vi "Read Sequence.vi"(8 "error in (no error)":errorcluster, 9 "Channel Mask":u64, 10 "Config Data":T3, 11 "Connection Data In":T2) -> (0 "error out":errorcluster, 1 "Adquisition Data Out":T1, 3 "Connection Data Out":T2)   [LabVIEW 2014, in "MSX-E3701_dll.lvlib"]
doc: "Recibe el Channel mask y el Config data. Abre el puerto e inicia la adquisición de valores en forma secuencial. Al mismo tiempo lee el estado de las I/O."
uses:
  MSX-E3701_dll.lvlib
  Typedef/Config Data.ctl
  Typedef/Connection Data.ctl
  E:/Repositorio Magnis/INF002/v0/Modules/HAL/Drivers/Sync/ADDI-DATA MSX-E3701/API/MX370x.dll
  MX370x.dll
  E:/Repositorio Magnis/INF002/v0/Modules/HAL/Drivers/Sync/ADDI-DATA MSX-E3701/API/MXCommon.dll
  MXCommon.dll
  Typedef/Adquisition Data.ctl
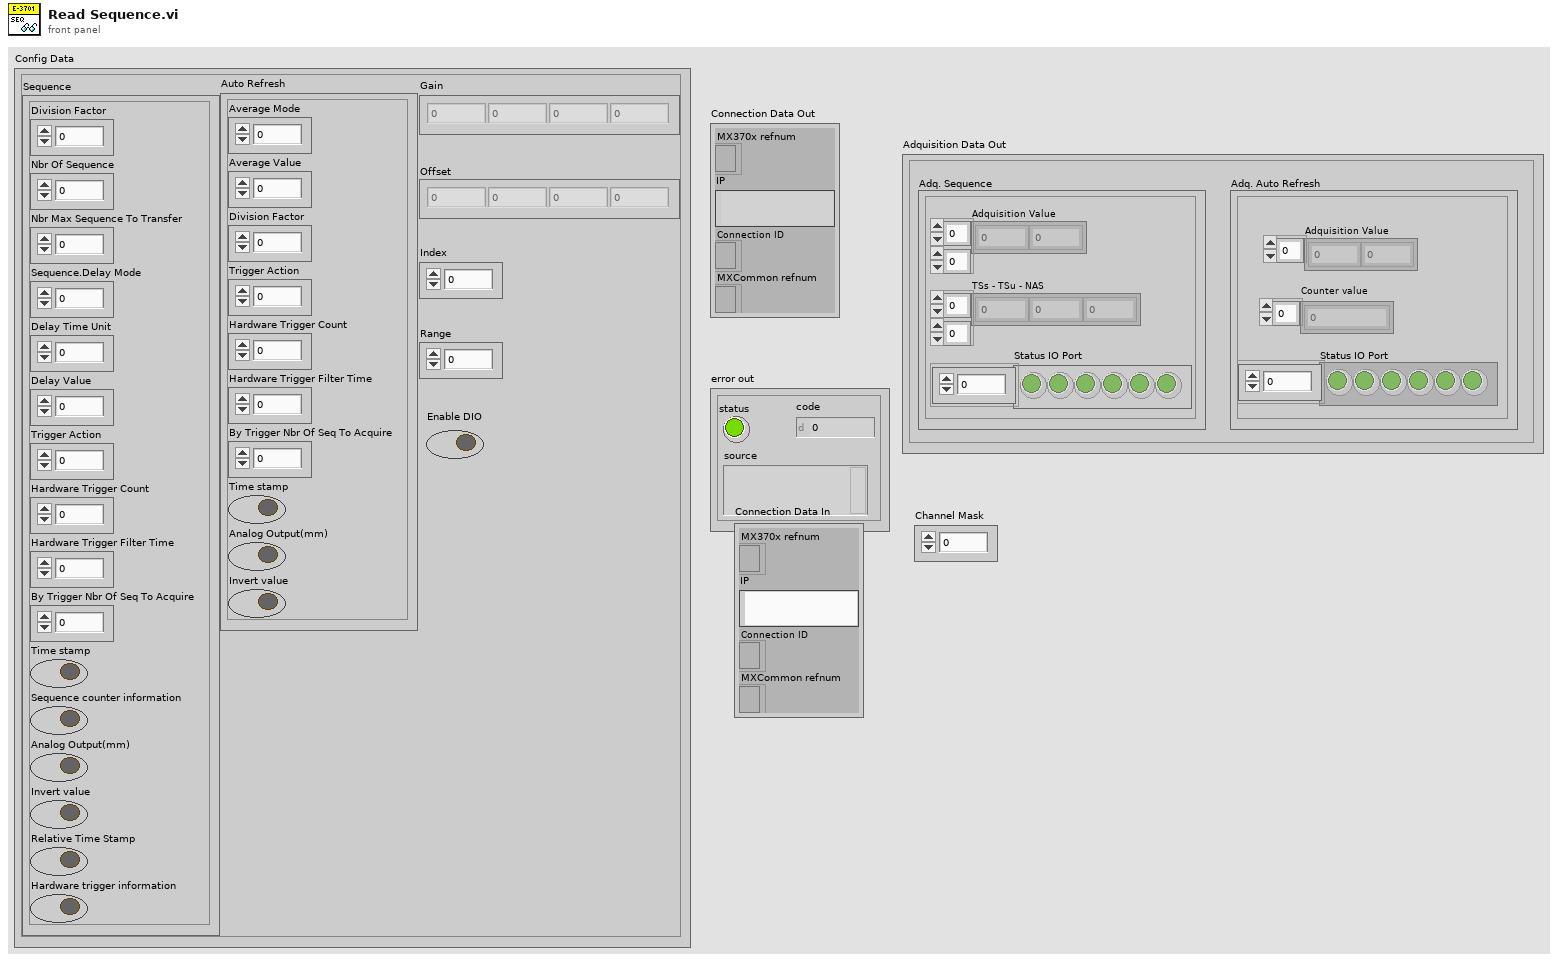
[diagram p1: front panel]
types:
  T1 = typedef "MSX-E3701_dll.lvlib/Adquisition Data.ctl" = cluster{"Adq. Sequence":cluster{"TSs - TSu - NAS":u64[][], "Adquisition Value":u32[][], "Status IO Port":bool[]}, "Adq. Auto Refresh":cluster{"Adquisition Value":u64[], "Status IO Port":bool[], "Counter value":u64[]}}
  T2 = typedef "MSX-E3701_dll.lvlib/Connection Data.ctl" = cluster{"MX370x refnum":refnum<k24>, "IP":string, "Connection ID ":refnum<k5>, "MXCommon refnum":refnum<k24>}
  T3 = typedef "MSX-E3701_dll.lvlib/Config Data.ctl" = cluster{"Auto Refresh":cluster{"Average Mode":u64, "Average Value":u64, "Division Factor":u64, "Trigger Action":u64, "Hardware Trigger Count":u64, "Hardware Trigger Filter Time":u64, "By Trigger Nbr Of Seq To Acquire":u64, "Time stamp":bool, "Analog Output(mm)":bool, "Invert value":bool}, "Gain":sgl[], "Offset":sgl[], "Index":u64, "Range":sgl, "Sequence":cluster{"Division Factor":u64, "Nbr Of Sequence":u64, "Nbr Max Sequence To Transfer":u64, "Sequence.Delay Mode":u64, "Delay Time Unit":u64, "Delay Value":u64, "Trigger Action":u64, "Hardware Trigger Count":u64, "Hardware Trigger Filter Time":u64, "By Trigger Nbr Of Seq To Acquire":u64, "Time stamp":bool, "Sequence counter information":bool, "Analog Output(mm)":bool, "Invert value":bool, "Relative Time Stamp":bool, "Hardware trigger information":bool}, "Enable DIO":bool}
  T4 = cluster{"Division Factor":u64, "Nbr Of Sequence":u64, "Nbr Max Sequence To Transfer":u64, "Sequence.Delay Mode":u64, "Delay Time Unit":u64, "Delay Value":u64, "Trigger Action":u64, "Hardware Trigger Count":u64, "Hardware Trigger Filter Time":u64, "By Trigger Nbr Of Seq To Acquire":u64, "Time stamp":bool, "Sequence counter information":bool, "Analog Output(mm)":bool, "Invert value":bool, "Relative Time Stamp":bool, "Hardware trigger information":bool}
  T5 = enum16{"big-endian, network order", "native, host order", "little-endian"}
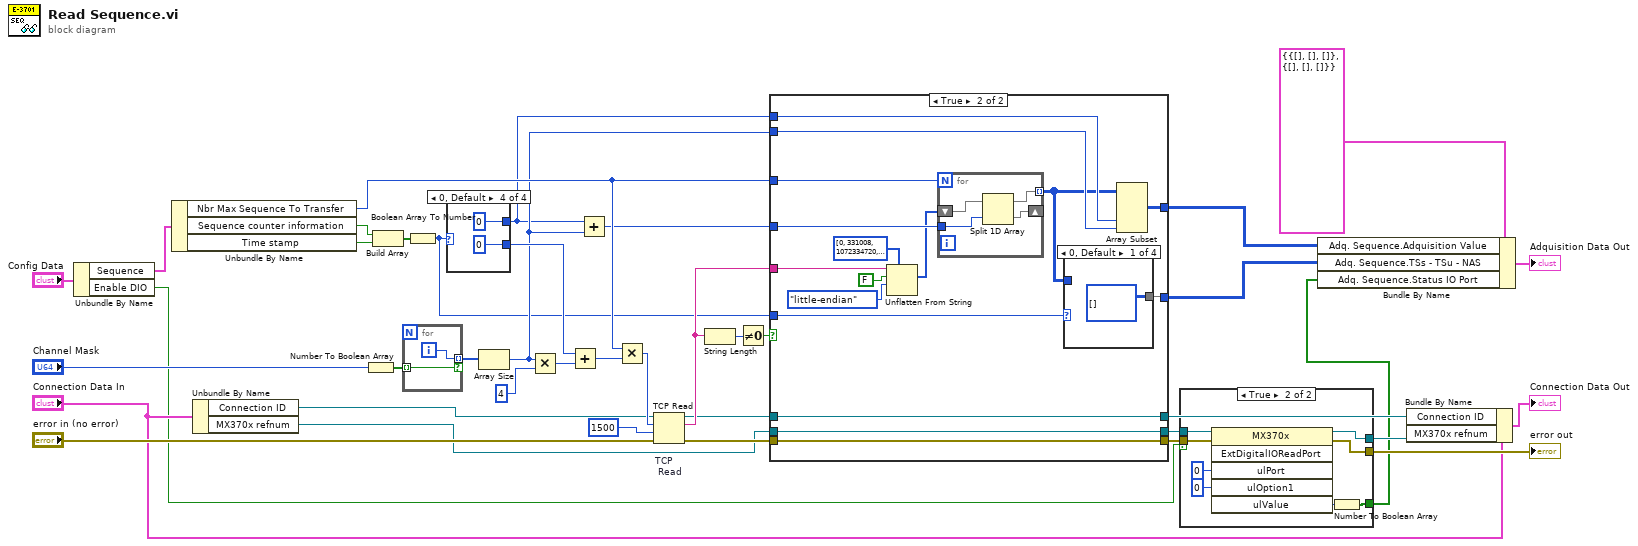
[diagram p0: block diagram]
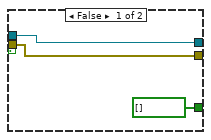
[diagram p2: hidden frame]
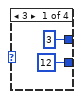
[diagram p3: hidden frame]
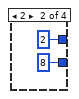
[diagram p4: hidden frame]
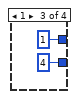
[diagram p5: hidden frame]
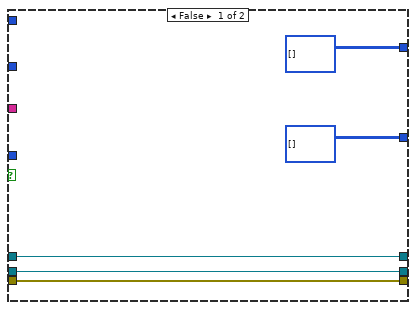
[diagram p6: hidden frame]
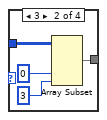
[diagram p7: hidden frame]
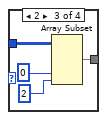
[diagram p8: hidden frame]
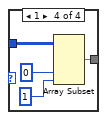
[diagram p9: hidden frame]
diagram:
  n1 = Unbundle By Name("Config Data") -> ("Sequence"=w37:T4, "Enable DIO"=w1:bool)
  n2 = Unbundle By Name(w37) -> ("Nbr Max Sequence To Transfer"=w14:u64, "Sequence counter information"=w13:bool, "Time stamp"=w12:bool)
  n3 = Unbundle By Name("Connection Data In") -> ("Connection ID"=w34:refnum<k5>, "MX370x refnum"=w18:refnum<k24>)
  n4 = Number To Boolean Array(number="Channel Mask") -> (Boolean array=w39:bool[])
  n5 = Build Array(w13, w12) -> (w11:bool[])
  n6 = for {
    tunnel: [w42] -> w38 mode=indexing if=w41
    tunnel: w39 -> [w41] mode=indexing
    i -> [w42]
  }
  n7 = Boolean Array To Number(Boolean array=w11) -> (number=w5:u32)
  n8 = case shown="0, Default" w5 {
    tunnel: [12 8 4 0] -> w10
    tunnel: [3 2 1 0] -> w7
    frame 3 {
    }
    frame 2 {
    }
    frame 1 {
    }
    frame 0, Default {
    }
  }
  n9 = Array Size(array=w38) -> (size(s)=w8:i32)
  n10 = Multiply(x=w8, y=4) -> (x*y=w6:i32)
  n11 = Add(x=w10, y=w6) -> (x+y=w36:i32)
  n12 = Add(x=w7, y=w8) -> (x+y=w9:i32)
  n13 = Multiply(x=w14, y=w36) -> (x*y=w35:u64)
  n14 = TCP Read "TCP\n Read"(connection ID=w34, bytes to read=w35, error in (no error)="error in (no error)", 9:1500 ("timeout ms (25000)")) -> (connection ID out=w21:refnum<k5>, data out=w26:string, error out=w25:errorcluster)  [unwired: 1 in]
  n15 = String Length(string=w26) -> (length=w28:i32)
  n16 = Not Equal To 0?(x=w28) -> (x != 0?=w27:bool)
  n17 = case shown="True" w27 {
    tunnel: w26 -> [_ w69]
    tunnel: w25 -> [w55 w68]
    tunnel: [w55 w68] -> w24
    tunnel: w14 -> [_ w56]
    tunnel: w9 -> [_ w67]
    tunnel: [w54 w66] -> w22
    tunnel: w21 -> [w54 w66]
    tunnel: w18 -> [w53 w65]
    tunnel: [w53 w65] -> w19
    tunnel: [u32[][] [] w64] -> w17
    tunnel: [u32[][] [] w60] -> w16
    tunnel: w8 -> [_ w62]
    tunnel: w7 -> [_ w61]
    tunnel: w5 -> [_ w58]
    frame False {
    }
    frame True {
      n18 = Unflatten From String(type=u32[] [0, 331008, 1072334720, 3195303168, 4729, 331808, 1072334336, 3195309312, 4729, 332608, 1072334080, 3195300096, 4729, 333408, 1072334400, 3195303936, 4729, 334208, 1072334336, 3195305728, 4729, 335008, 1072334400, 3195309568, 4729, 335808, 1072334912, 3195305472, 4729, 336608, 1072333568, 3195304704, 4729, 337408, 1072333440, 3195311872, 4729, 338208, 1072334720, 3195307264, 4729, 339008, 1072334272, 3195311616, 4729, 339808, 1072334272, 3195305984, 4729, 340608, 1072334400, 3195307776, 4729, 341408, 1072334080, 3195308288, 4729, 342208, 1072334720, 3195304448, 4729, 343008, 1072335488, 3195307264, 4729, 343808, 1072334080, 3195302912, 4729, 344608, 1072334272, 3195311360, 4729, 345408, 1072334848, 3195309056, 4729, 346208, 1072334784, 3195301376, 4729, 347008, 1072335168, 3195305472, 4729, 347808, 1072334912, 3195314688, 4729, 348608, 1072334080, 3195299584, 4729, 349408, 1072334144, 3195304448, 4729, 350208, 1072334400, 3195304448, 4729, 351008, 1072335296, 3195304960, 4729, 351808, 1072334144, 3195309824, 4729, 352608, 1072334784, 3195303168, 4729, 353408, 1072334464, 3195305472, 4729, 354208, 1072335168, 3195313920, 4729, 355008, 1072334400, 3195304960, 4729, 355808, 1072334144, 3195304192, 4729, 356608, 1072334528, 3195307776, 4729, 357408, 1072335104, 3195309056, 4729, 358208, 1072333824, 3195308544, 4729, 359008, 1072334208, 3195309312, 4729, 359808, 1072334272, 3195306240, 4729, 360608, 1072334848, 3195309312, 4729, 361408, 1072334656, 3195302912, 4729, 362208, 1072334528, 3195305216, 4729, 363008, 1072334528, 3195304192, 4729, 363808, 1072335232, 3195316480, 4729, 364608, 1072334784, 3195305216, 4729, 365408, 1072333824, 3195308800, 4729, 366208, 1072334784, 3195309312, 4729, 367008, 1072334784, 3195302656, 4729, 367808, 1072333632, 3195310336, 4729, 368608, 1072333568, 3195305984, 4729, 369408, 1072334336, 3195305728, 4729, 370208, 1072334656, 3195304448, 4729, 371008, 1072334208, 3195305984, 4729, 371808, 1072334336, 3195306240, 4729, 372608, 1072334144, 3195302656, 4729, 373408, 1072334592, 3195300864, 4729, 374208, 1072334016, 3195302400, 4729, 375008, 1072334144, 3195307264, 4729, 375808, 1072334528, 3195312640, 4729, 376608, 1072334784, 3195302400, 4729, 377408, 1072333696, 3195305728, 4729, 378208, 1072334656, 3195302144, 4729, 379008, 1072334464, 3195306752, 4729, 379808, 1072334272, 3195306496, 4729, 380608, 1072334272, 3195307776, 4729, 381408, 1072334400, 3195306496, 4729, 382208, 1072334592, 3195300608, 4729, 383008, 1072334400, 3195303168, 4729, 383808, 1072334016, 3195304192, 4729, 384608, 1072334016, 3195309568, 4729, 385408, 1072334912, 3195306496, 4729, 386208, 1072334656, 3195303424, 4729, 387008, 1072334080, 3195302912, 4729, 387808, 1072334592, 3195309312, 4729, 388608, 1072334272, 3195299072, 4729, 389408, 1072334144, 3195304704, 4729, 390208, 1072334272, 3195304960, 4729, 391008, 1072334144, 3195305472, 4729, 391808, 1072334336, 3195301632, 4729, 392608, 1072334464, 3195307008, 4729, 393408, 1072334016, 3195311616, 4729, 394208, 1072335168, 3195310336, 4729, 395008, 1072335232, 3195308288, 4729, 395808, 1072334592, 3195303680, 4729, 396608, 1072334016, 3195308288, 4729, 397408, 1072335296, 3195304448, 4729, 398208, 1072334400, 3195310080, 4729, 399008, 1072334464, 3195302912, 4729, 399808, 1072334848, 3195305728, 4729, 400608, 1072334464, 3195306752, 4729, 401408, 1072334272, 3195306240, 4729, 402208, 1072334656, 3195305216, 4729, 403008, 1072334272, 3195307008, 4729, 403808, 1072335296, 3195315968, 4729, 404608, 1072334336, 3195302656, 4729, 405408, 1072334336, 3195304192, 4729, 406208, 1072334528, 3195309568, 4729, 407008, 1072334912, 3195303168, 4729, 407808, 1072333952, 3195309312, 4729, 408608, 1072334272, 3195307520, 4729, 409408, 1072334464, 3195306496, 4729, 410208, 1072334400, 3195305472] ("Array - Numeric"), binary string=w69, data includes array or string size? (T)=FALSE, byte order (0:big-endian, network order)=T5."little-endian") -> (value=w63:u32[])  [unwired: 1 in, 2 out]
      n19 = for {
        N: w56 -> [_]
        shift-right: [w85] -> _
        shift-left: w63 -> [w88]
        tunnel: [w87] -> w59 mode=indexing
        tunnel: w67 -> [w86]
        n20 = Split 1D Array(array=w88, index=w86) -> (first subarray=w87:u32[], second subarray=w85:u32[])
      }
      n21 = case shown="0, Default" w58 {
        tunnel: [u64[][] [] w75 w79 w84] -> w60
        tunnel: w59 -> [_ w76 w80 w83]
        frame 0, Default {
        }
        frame 3 {
          n22 = Array Subset(array=w76, index (col)=0 ("index"), length (col)=3 ("length")) -> (w75:u32[][])  [unwired: 2 in]
        }
        frame 2 {
          n23 = Array Subset(array=w80, index (col)=0 ("index"), length (col)=2 ("length")) -> (w79:u32[][])  [unwired: 2 in]
        }
        frame 1 {
          n24 = Array Subset(array=w83, index (col)=0 ("index"), length (col)=1 ("length")) -> (w84:u32[][])  [unwired: 2 in]
        }
      }
      n25 = Array Subset(array=w59, index (col)=w61, length (col)=w62) -> (w64:u32[][])  [unwired: 2 in]
    }
  }
  n26 = case shown="True" w1 {
    tunnel: [w89 w99] -> w31
    tunnel: w24 -> [w89 w98]
    tunnel: [w90 w97] -> w20
    tunnel: w19 -> [w90 w96]
    tunnel: [bool[] [] ("Boolean array") w92] -> w3
    frame False {
    }
    frame True {
      n27 = invoke class="MX370x" method="ExtDigitalIOReadPort"(reference=w96, error in=w98, "ulPort"=u64 0, "ulOption1"=u64 0) -> (reference out=w97:refnum<k24>, error out=w99:errorcluster, "ulValue"=w95:u64)  [unwired: 2 in, 3 out]
      n28 = Number To Boolean Array(number=w95) -> (Boolean array=w92:bool[])
    }
  }
  "error out" <- w31
  n29 = Bundle By Name(cluster=T1 {"Adq. Sequence"={"TSs - TSu - NAS"=[], "Adquisition Value"=[], "Status IO Port"=[]}, "Adq. Auto Refresh"={"Adquisition Value"=[], "Status IO Port"=[], "Counter value"=[]}} ("Adquisition Data In"), "Adq. Sequence.Adquisition Value"=w17, "Adq. Sequence.TSs - TSu - NAS"=w16, "Adq. Sequence.Status IO Port"=w3) -> (→"Adquisition Data Out":T1)
  n30 = Bundle By Name(cluster="Connection Data In", "Connection ID"=w22, "MX370x refnum"=w20) -> (→"Connection Data Out":T2)
